vi "example (factorial).vi"() -> ()   [LabVIEW 2021]
panel:
  in  "stop":bool
  out "Factorial":dbl
  in  "n":dbl
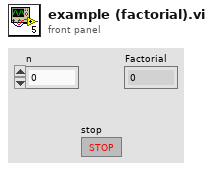
[diagram p1: front panel]
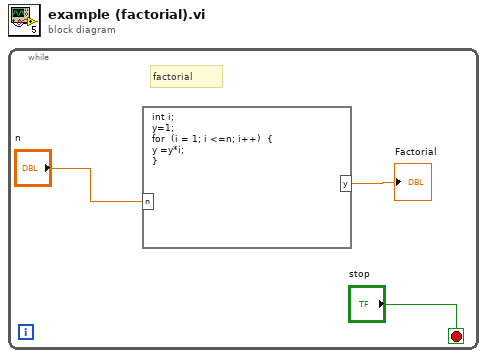
[diagram p0: block diagram]
diagram:
  n1 = while {
    stop <- "stop" stop-if-true
    # "factorial"
    n2 = formula code="int i;\ny=1;\nfor  (i = 1; i <=n; i++)  {\ny =y*i;\n}"("n"="n") -> ("y"=→"Factorial":dbl)
  }
